vi "Receive.vi"(8 "error in (no error)":errorcluster caption="错误输入（无错误）", 11 "ZLGCAN 输入":refnum<class "ZLGCAN.lvclass">) -> (0 "error out":errorcluster caption="错误输出", 2 "数组":T1[](array[typedef]) {"Data" format="%x"; "ID" format="%x"}, 3 "ZLGCAN 输出":refnum<class "ZLGCAN.lvclass">)   [LabVIEW 2020, in "ZLGCAN.lvclass"]
uses:
  ZLGCAN.lvclass
  CAN/CANData.ctl
  ZLGCAN.lvclass/ZLGCAN.ctl
  CAN/CAN.lvclass
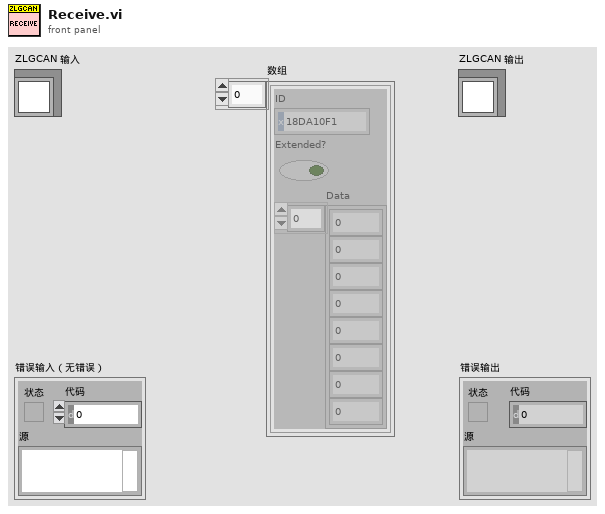
[diagram p1: front panel]
types:
  T1 = typedef "CAN.lvclass/CANData.ctl" = cluster{"ID":u32, "Extended?":bool, "Data":u8[]}
  T2 = cluster{"Device Type":u32, "Device Index":u32, "CANInd":u32, "Baud(E_U)":u32}
  T3 = typedef "ZLGCAN.lvclass/VCI_CAN_OBJ.ctl" = cluster{"ID":u32, "TimeStamp":u32, "TimeFlag":enum8{"invalid", "valid"}, "SendType":enum8{"Normal", "Once", "Test", "Once Test"}, "RemoteFlag":enum8{"Data", "Remote"}, "ExternFlag":enum8{"Standard", "Extern"}, "DataLen":u8, "Data0":u8, "Data1":u8, "Data2":u8, "Data3":u8, "Data4":u8, "Data5":u8, "Data6":u8, "Data7":u8, "Reserved0":u8, "Reserved1":u8, "Reserved2":u8}
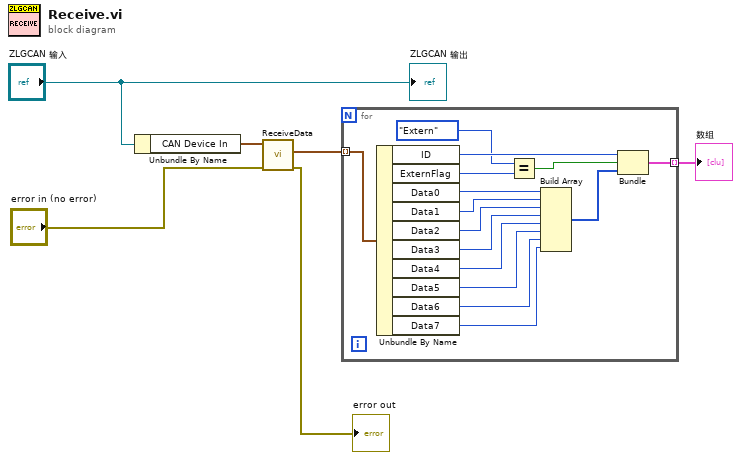
[diagram p0: block diagram]
diagram:
  n1 = Unbundle By Name("ZLGCAN 输入") -> ("CAN Device In"=w5:T2)
  n2 = call "ReceiveData.vi"("Error In(No Error)"="error in (no error)", "CAN Device In"=w5) -> ("Error Out"=→"error out":errorcluster, "pReceive"=w4:T3[])  [unwired: 6 in, 2 out]
  n3 = for {
    tunnel: w4 -> [w21] mode=indexing
    tunnel: [w10] -> w3 mode=indexing
    n4 = Unbundle By Name(w21) -> ("ID"=w12:u32, "ExternFlag"=w8:enum8{"Standard", "Extern"}, "Data0"=w20:u8, "Data1"=w19:u8, "Data2"=w18:u8, "Data3"=w17:u8, "Data4"=w16:u8, "Data5"=w15:u8, "Data6"=w14:u8, "Data7"=w13:u8)
    n5 = Equal?(x=enum8{"Standard", "Extern"}."Extern" ("y"), y=w8) -> (x = y?=w7:bool)
    n6 = Build Array(w20, w19, w18, w17, w16, w15, w14, w13) -> (w11:u8[])
    n7 = Bundle("ID"=w12, w7, w11) -> (w10:cluster{"ID":u32, bool, u8[]})  [unwired: 1 in]
  }
  "数组" <- w3
  "ZLGCAN 输出" <- "ZLGCAN 输入"
